vi "Set SG Path.vi"(0 "Path in":refnum<class "SG 18GHz Path.lvclass">, 5 "Cal point in":T1, 11 "error in":errorcluster) -> (4 "Path out":refnum<class "SG 18GHz Path.lvclass">, 6 "Cal point out":T1, 8 "Source Gain":dbl, 10 "Digital Gain":dbl, 15 "error out":errorcluster)   [LabVIEW 2023, in "RFFixtureCharact.RFPM.lvlib" / "SG 18GHz Path.lvclass"]
uses:
  SG 18GHz Path.lvclass
  Public/Base Classes/Scalar/Scalar Path/Type Definitions/Cal Point.ctl
  C:/srd-semi-rfcal-software/AuxTools/STSRFFixtureCharactUtility/Source/Code Modules/Common/Base Classes/Path/Path.lvclass
  <instrlib>/niRFPM/niRFPM.llb/NI-RFPM Set TX Path By Switch Path String.vi
  Public/Base Classes/Scalar/Scalar Path/Scalar Path.lvclass
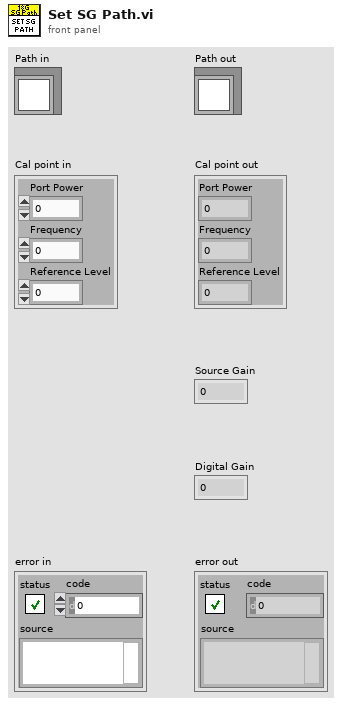
[diagram p1: front panel]
types:
  T1 = typedef "RFFixtureCharact.Public.lvlib/Scalar Path.lvclass/Cal Point.ctl" = cluster{"Port Power":dbl, "Frequency":dbl, "Reference Level":dbl}
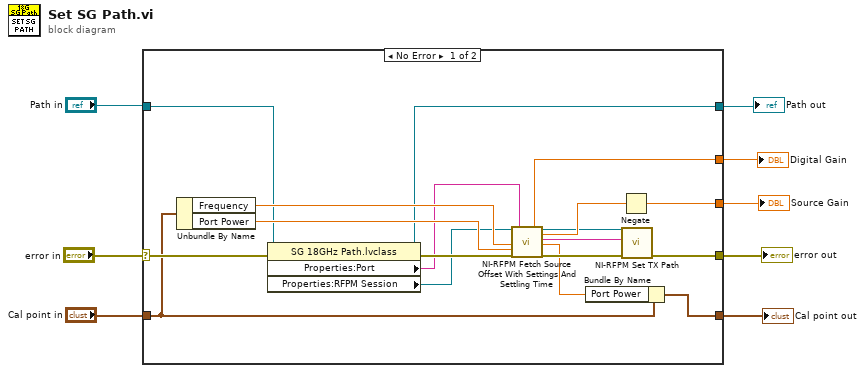
[diagram p0: block diagram]
diagram:
  n1 = case shown="No Error" "error in" {
    selector: "error in" -> [w17 w29]
    tunnel: [w18 w29] -> w4
    tunnel: [w15 w28] -> w1
    tunnel: "Path in" -> [w16 w28]
    tunnel: [w19 _] -> w3
    tunnel: "Cal point in" -> [w12 w27]
    tunnel: [w10 w27] -> w5
    tunnel: [w9 _] -> w2
    frame No Error {
      n2 = Unbundle By Name(w12) -> ("Frequency"=w26:dbl, "Port Power"=w25:dbl)
      n3 = property class="SG 18GHz Path.lvclass"(reference=w16, error in=w17) -> (reference out=w15:refnum<class "SG 18GHz Path.lvclass">, error out=w24:errorcluster, "Properties:Port"=w14:string, "Properties:RFPM Session"=w13:refnum<k15>)
      n4 = call <instrlib>:"NI-RFPM Fetch Source Offset With Settings And Settling Time.vi"("instrument handle"=w13, "Frequency"=w26, "Power"=w25, "error in"=w24, "Port"=w14) -> ("Digital Gain"=w9:dbl, "instrument handle out"=w20:refnum<k15>, "Source Offset"=w23:dbl, "Switch Path String"=w22:string, "Calibrated Power"=w11:dbl, "error out"=w21:errorcluster)  [unwired: 8 in, 1 out]
      n5 = Bundle By Name(cluster=w12, "Port Power"=w11) -> (w10:T1)
      n6 = Negate(x=w23) -> (-x=w19:dbl)
      n7 = call-poly <instrlib>:"NI-RFPM Set TX Path.vi"("instrument handle"=w20, "TX Switch Path"=w22, "error in (no error)"=w21) -> ("error out"=w18:errorcluster)  [unwired: 11 in, 1 out]
    }
    frame Error {
    }
  }
  "error out" <- w4
  "Source Gain" <- w3
  "Cal point out" <- w5
  "Digital Gain" <- w2
  "Path out" <- w1
